vi "Write Key (String).vi"(6 "write raw string? (F)":bool, 7 "section":string, 8 "error in (no error)":errorcluster, 9 "value":string, 10 "key":string, 11 "refnum":T1) -> (0 "error out":errorcluster, 2 "found?":bool, 3 "refnum out":T1)   [LabVIEW 2017, in "NI_LVConfig.lvlib"]
doc: "Writes a value to a key in a specified section of the configuration data identified by <B>refnum</B>. This VI modifies data in memory. To write data to disk, use the Close Config Data VI. Wire data to the <B>value</B> input to determine the polymorphic instance to use or manually select the instance."
uses:
  <vilib>/Utility/config.llb/NI_LVConfig.lvlib
  <vilib>/Utility/config.llb/Config Data RefNum.ctl
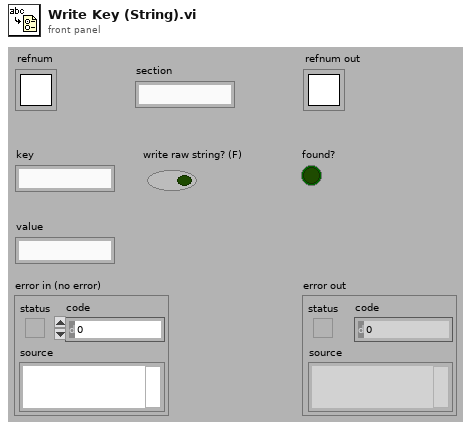
[diagram p1: front panel]
types:
  T1 = typedef "NI_LVConfig.lvlib/Config Data RefNum.ctl" = refnum<k1>
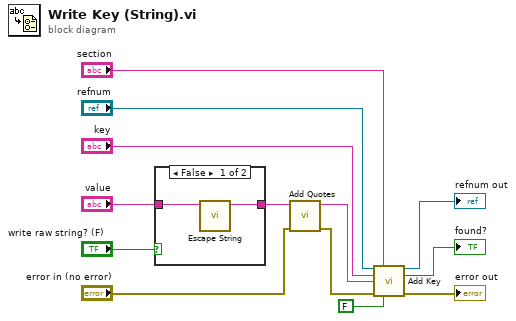
[diagram p0: block diagram]
diagram:
  n1 = case shown="False" "write raw string? (F)" {
    tunnel: "value" -> [w15 w16]
    tunnel: [w14 w16] -> w4
    frame False {
      n2 = call <vilib>:"Escape String.vi"("input"=w15) -> ("output"=w14:string)  [unwired: 10 in]
    }
    frame True {
    }
  }
  n3 = call <vilib>:"Add Quotes.vi"("error in (no error)"="error in (no error)", "string"=w4) -> ("error out"=w1:errorcluster, "with quotes"=w3:string)  [unwired: 8 in]
  n4 = call <vilib>:"Add Key.vi"("refnum"="refnum", "section"="section", "key"="key", "value"=w3, "error in (no error)"=w1, "add comment"=FALSE) -> ("refnum out"=→"refnum out":T1, "key exists?"=→"found?":bool, "error out"=→"error out":errorcluster)  [unwired: 7 out]
